vi "string.vi"() -> ()   [LabVIEW 2019]
panel:
  out "array":dbl[][](array[numeric])
  out "spreadsheet string":string
  out "number":dbl
  out "F-format string":string
  out "String":string
  out "concatenated string":string
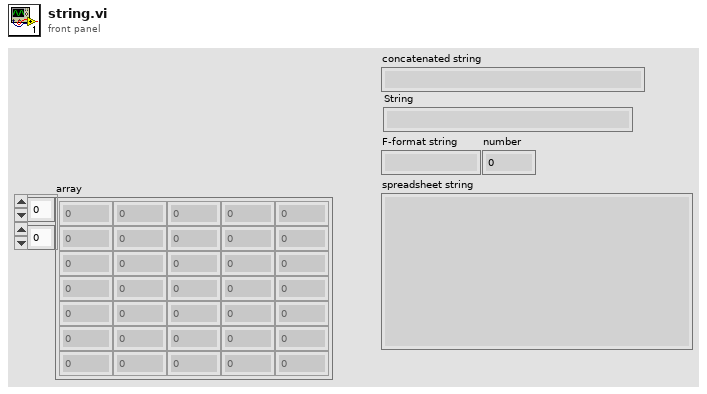
[diagram p1: front panel]
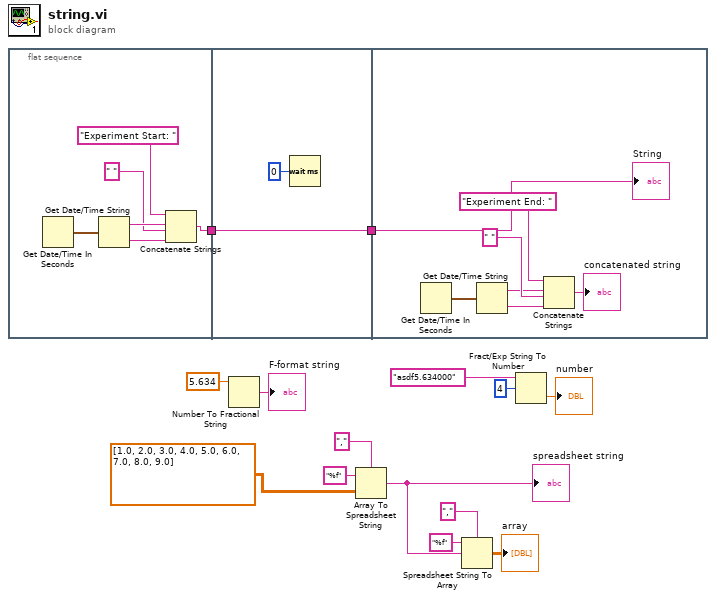
[diagram p0: block diagram]
diagram:
  n1 = flat-sequence {
    tunnel: [w16] -> w14
    tunnel: w14 -> [w21]
    tunnel: [w21] -> w13
    tunnel: w13 -> [w23]
    frame #0 {
      n2 = Get Date/Time In Seconds() -> (seconds since 1Jan1904=w20:timestamp)
      n3 = Get Date/Time String(seconds (now)=w20) -> (date string=w19:string, time string=w18:string)  [unwired: 2 in]
      n4 = Concatenate Strings("Experiment Start: " ("string"), w19, " " ("string"), w18) -> (w16:string)
    }
    frame #1 {
      n5 = Wait (ms)(milliseconds to wait=u32 0) -> ()  [unwired: 1 out]
    }
    frame #2 {
      n6 = Get Date/Time In Seconds() -> (seconds since 1Jan1904=w25:timestamp)
      n7 = Get Date/Time String(seconds (now)=w25) -> (date string=w26:string, time string=w27:string)  [unwired: 2 in]
      n8 = Concatenate Strings("Experiment End: " ("string"), w26, " " ("string"), w27) -> (→"concatenated string":string)
      "String" <- w23
    }
  }
  n9 = Number To Fractional String(number=5.634) -> (F-format string=→"F-format string":string)  [unwired: 3 in]
  n10 = Array To Spreadsheet String(delimiter (Tab)=",", array=dbl[][] [[1.0, 2.0, 3.0], [4.0, 5.0, 6.0], [7.0, 8.0, 9.0]], 3:"%f" ("format string")) -> (spreadsheet string=w4:string)
  "spreadsheet string" <- w4
  n11 = Spreadsheet String To Array(delimiter (Tab)=",", format string="%f", spreadsheet string=w4) -> (array=→"array":dbl[][])  [unwired: 1 in]
  n12 = Fract/Exp String To Number(string="asdf5.634000" ("F-format string 2"), offset=4) -> (number=→"number":dbl)  [unwired: 2 in, 1 out]
